vi "xcorr bkp nico.vi"(4 "shift":u8, 6 "N":u8, 7 "y":u32, 8 "x":u32, 9 "enable":bool, 10 "lag":u16) -> (1 "Rxy valid":bool, 2 "Rxy":u64, 3 "trigger":bool)   [LabVIEW 2017]
uses:
  <vilib>/rvi/FXPMathLib/basic elements/FxpDiscreteDelay/XNode/nifxpmath_DiscreteDelay.xnode
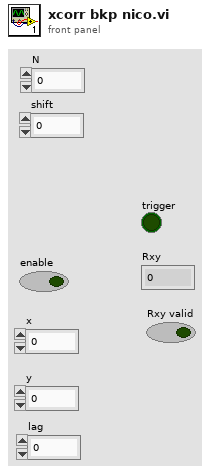
[diagram p1: front panel]
types:
  T1 = cluster{"Q":bool, "Q":bool, "Q":bool, "Q":bool, "valid":bool}
  T2 = cluster{"Q":bool, "Q":bool, "Q":bool, "Q":bool, "Q":bool, "Q":bool, "valid":bool}
  T3 = cluster{"Q":bool, "Q":bool, "Q":bool, "Q":bool, "Q":bool, "Q":bool, "Q":bool, "Q":bool, "Q":bool, "Q":bool, "Q":bool, "Q":bool, "valid":bool}
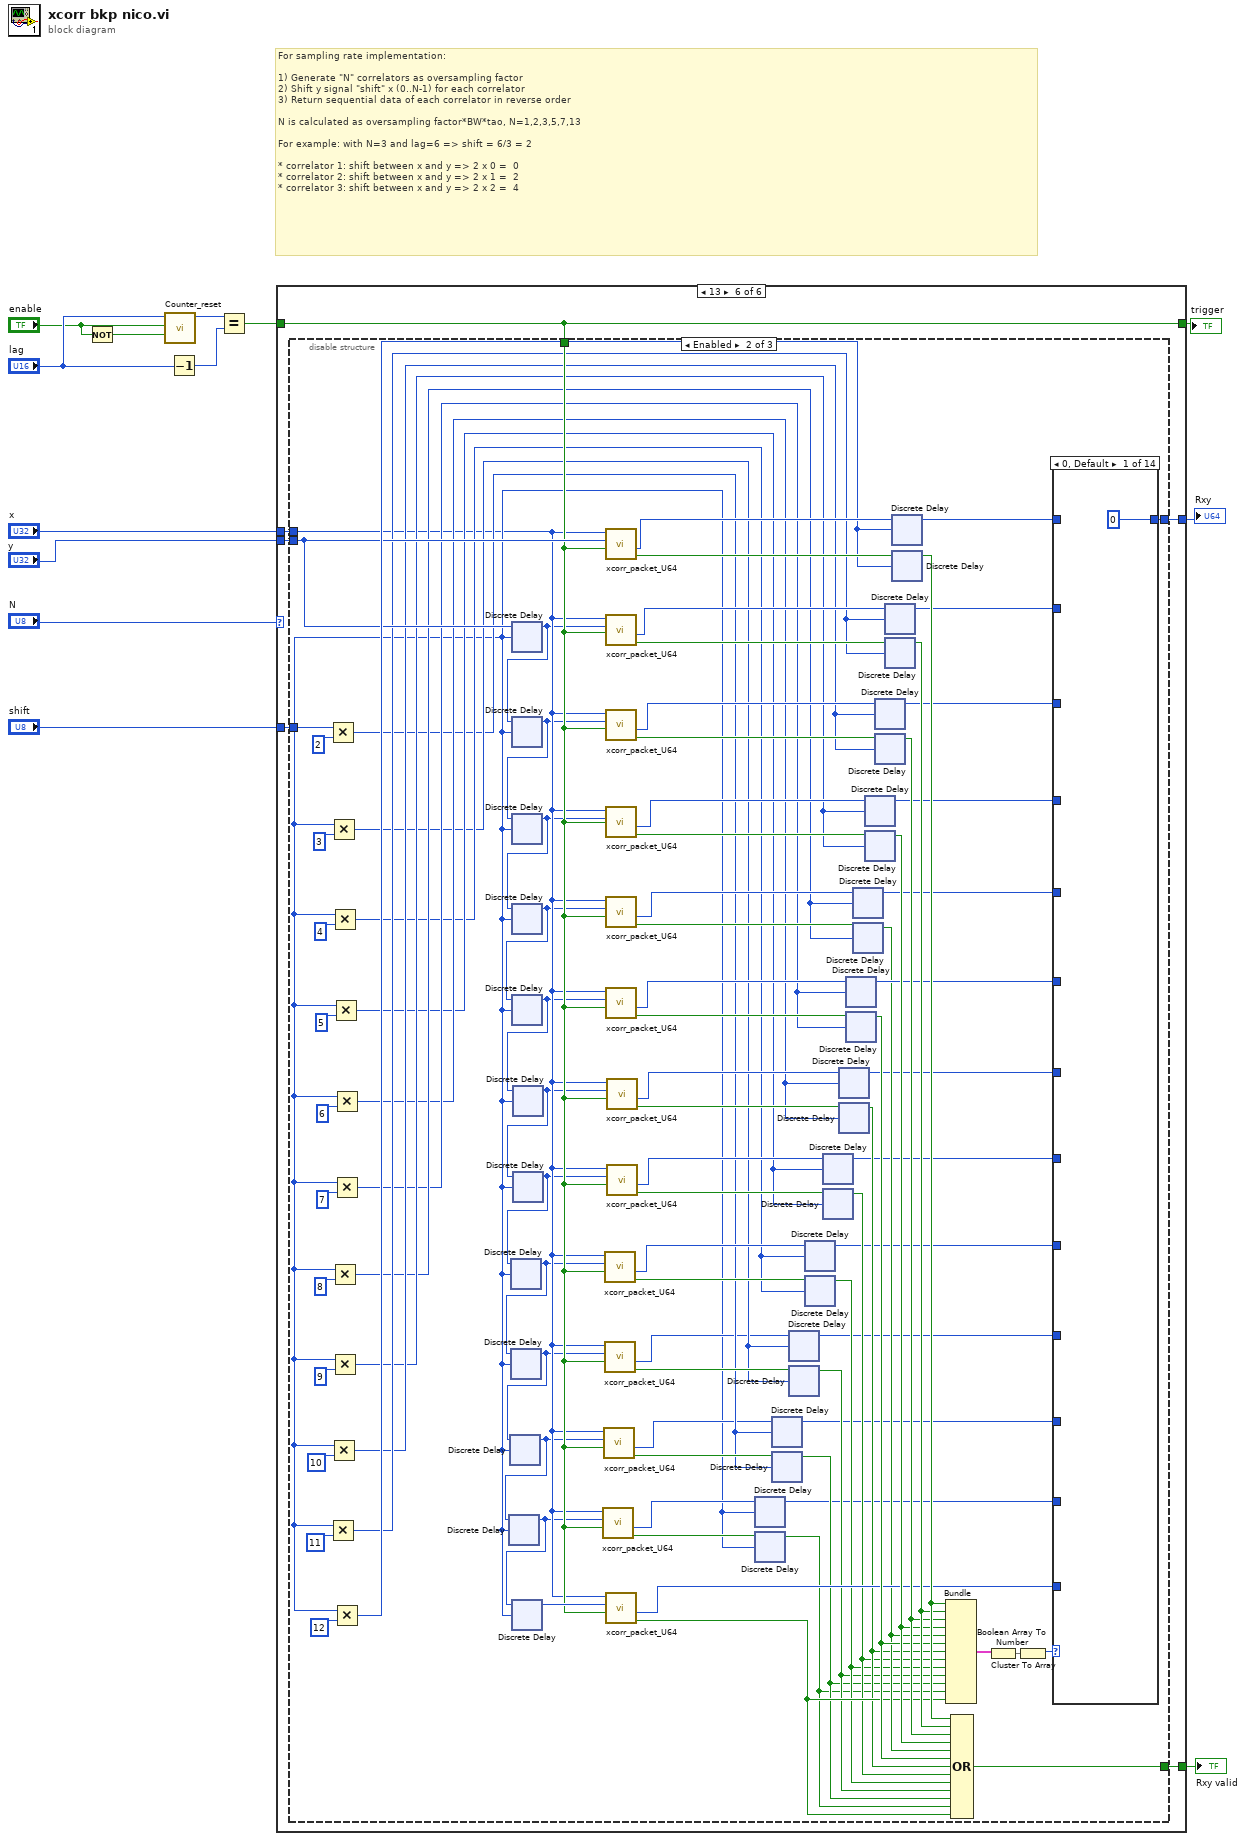
[diagram p0: block diagram]
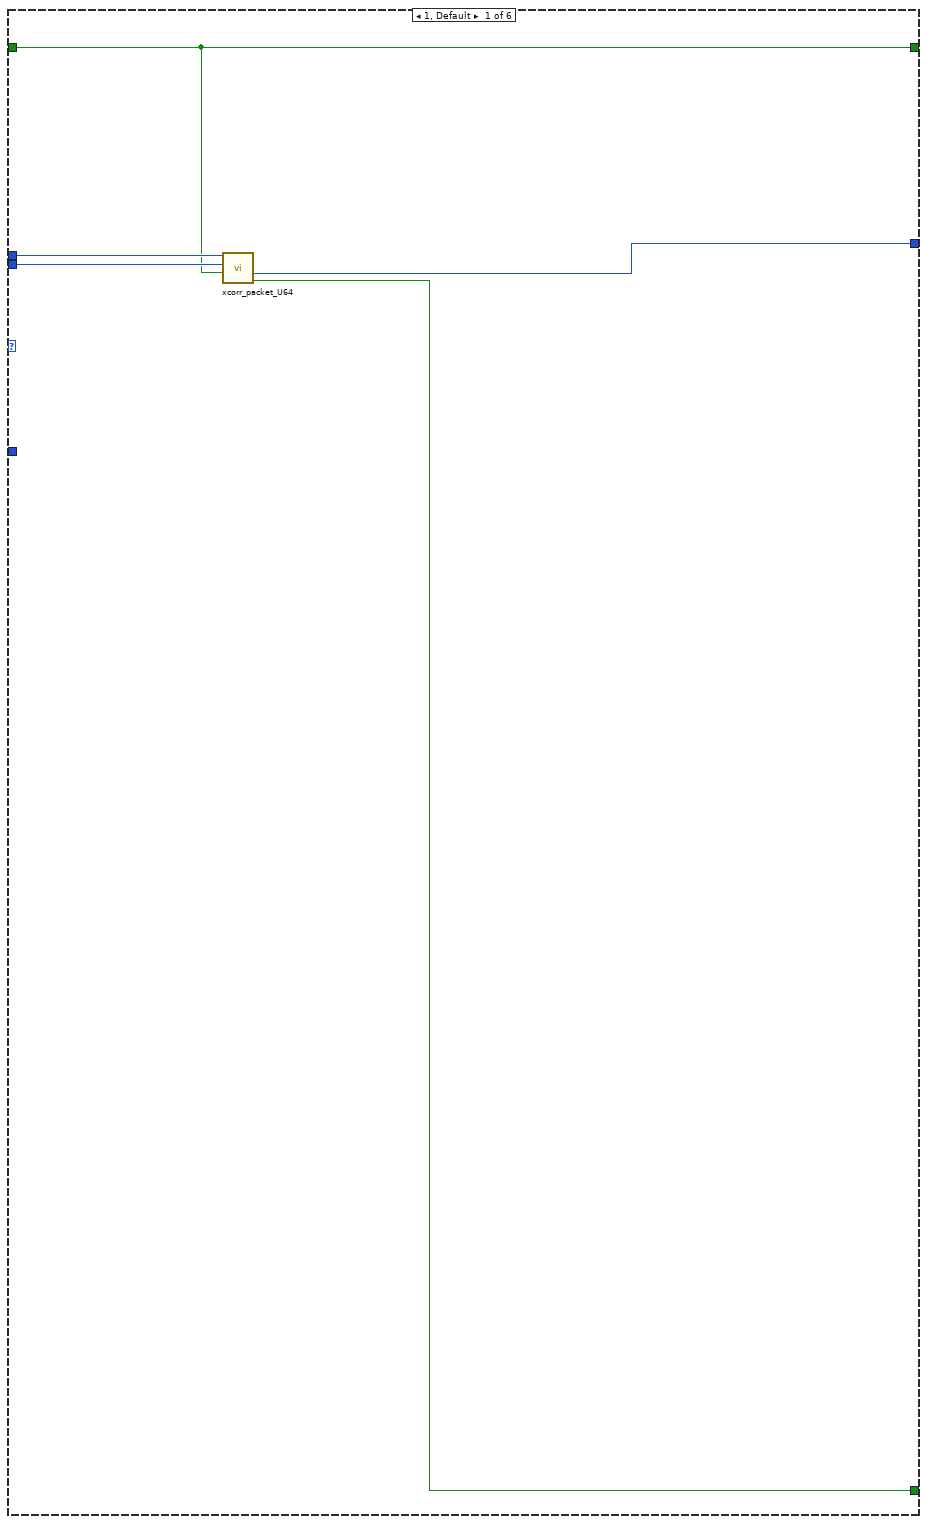
[diagram p2: hidden frame]
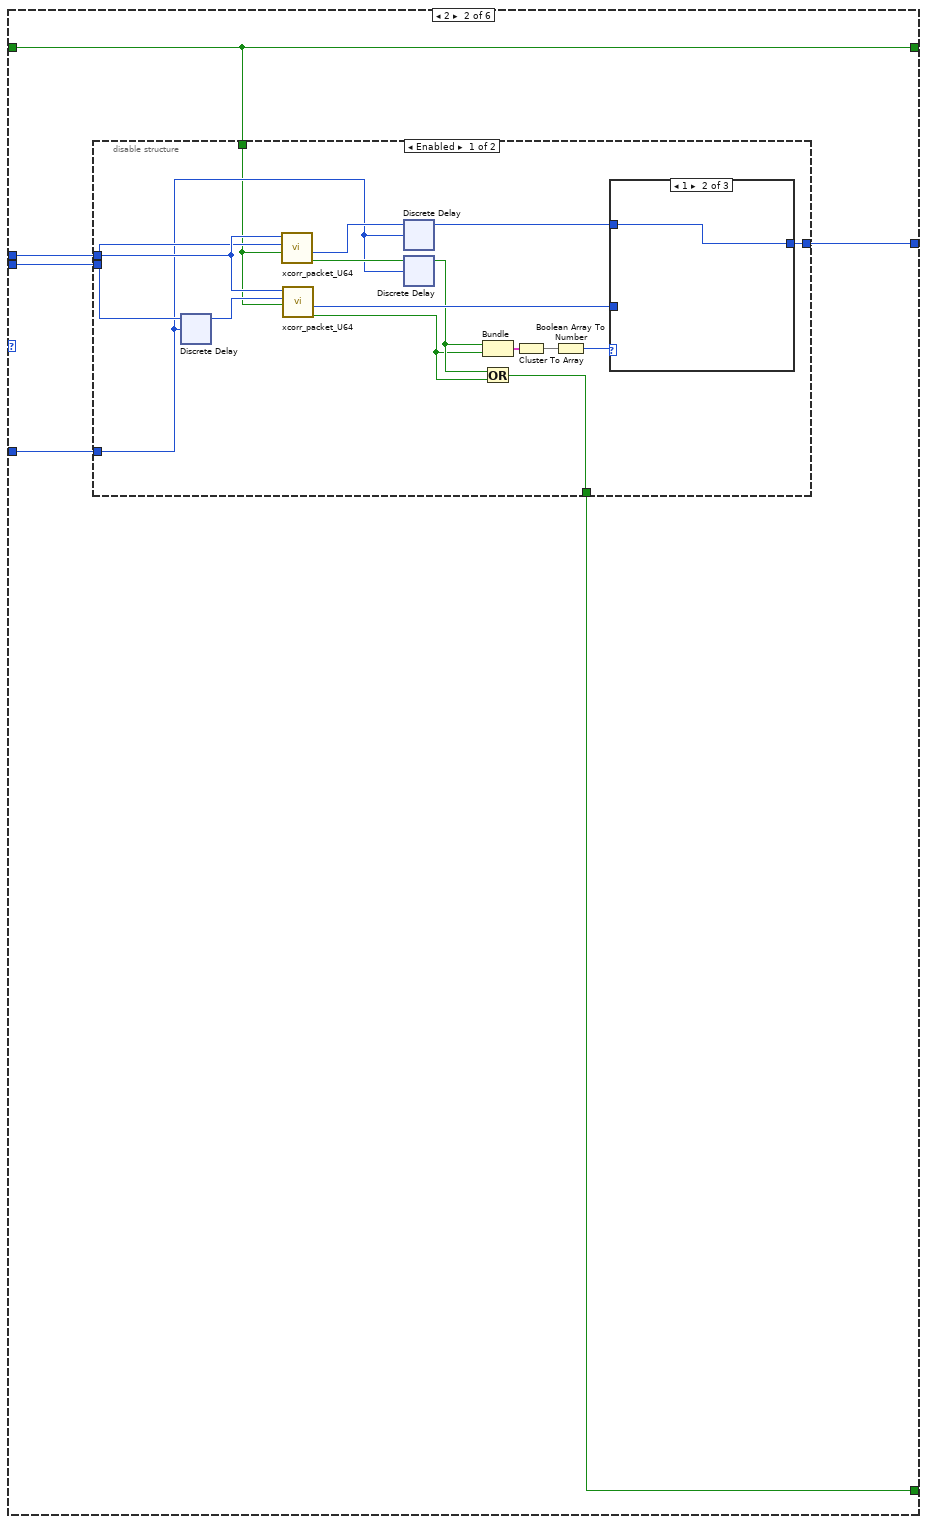
[diagram p3: hidden frame]
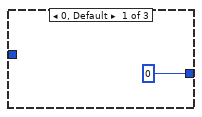
[diagram p4: hidden frame]
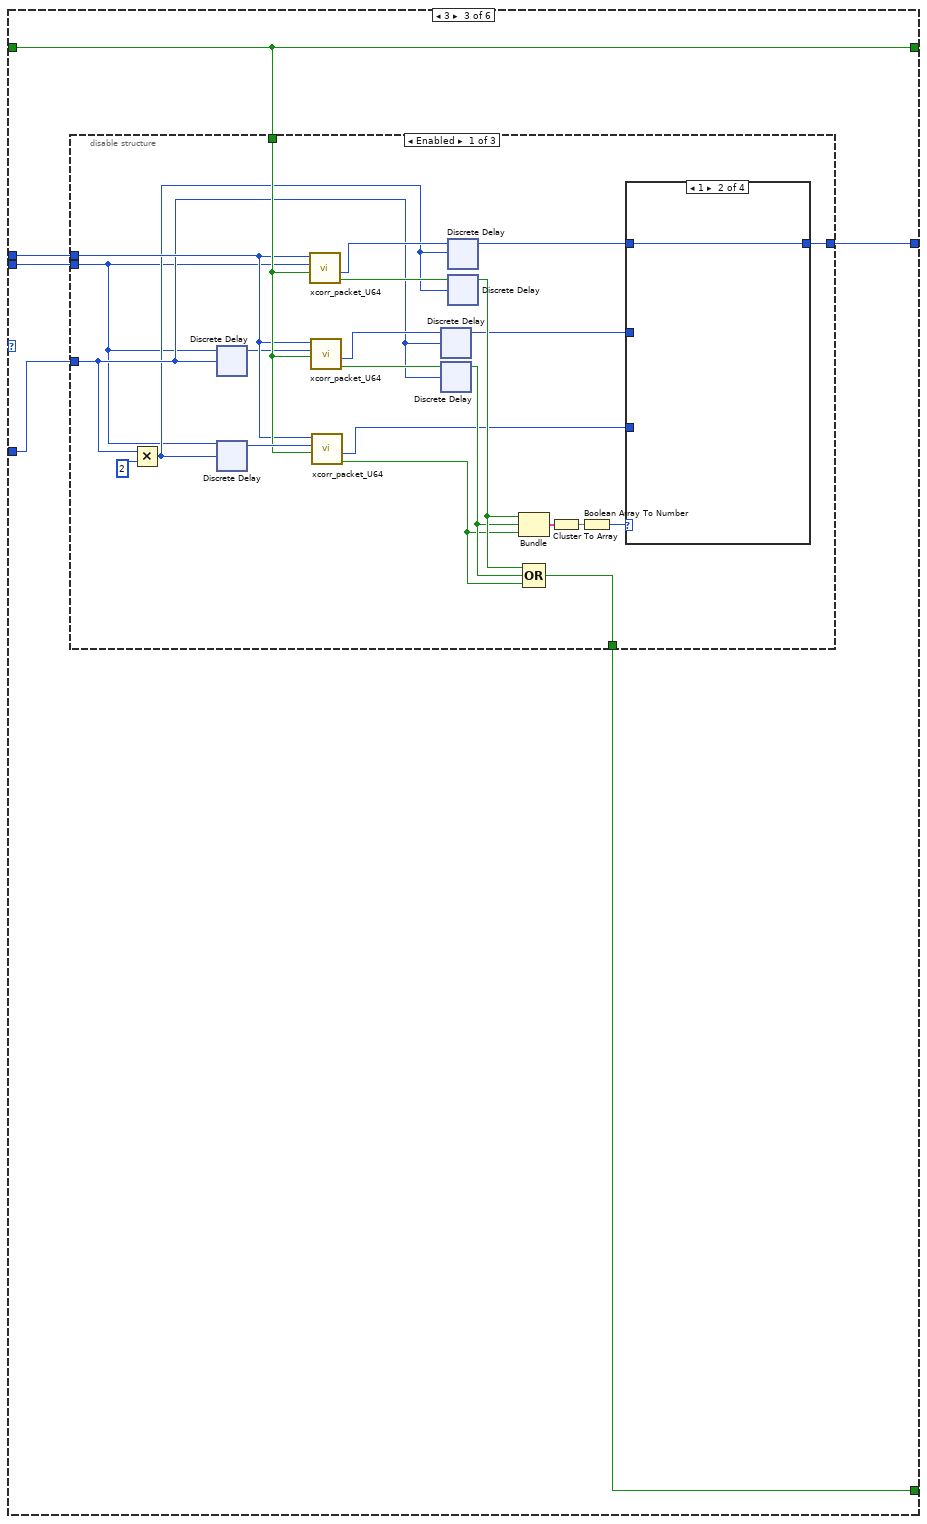
[diagram p7: hidden frame]
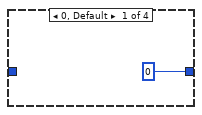
[diagram p8: hidden frame]
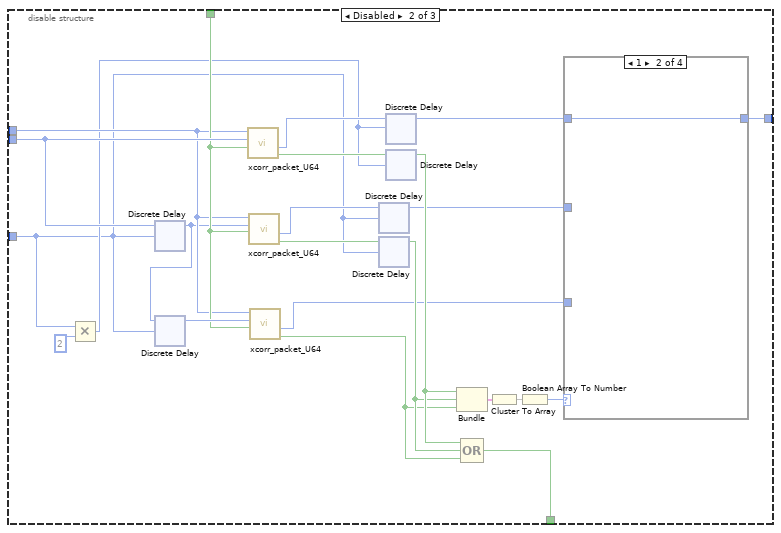
[diagram p11: hidden frame]
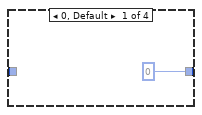
[diagram p12: hidden frame]
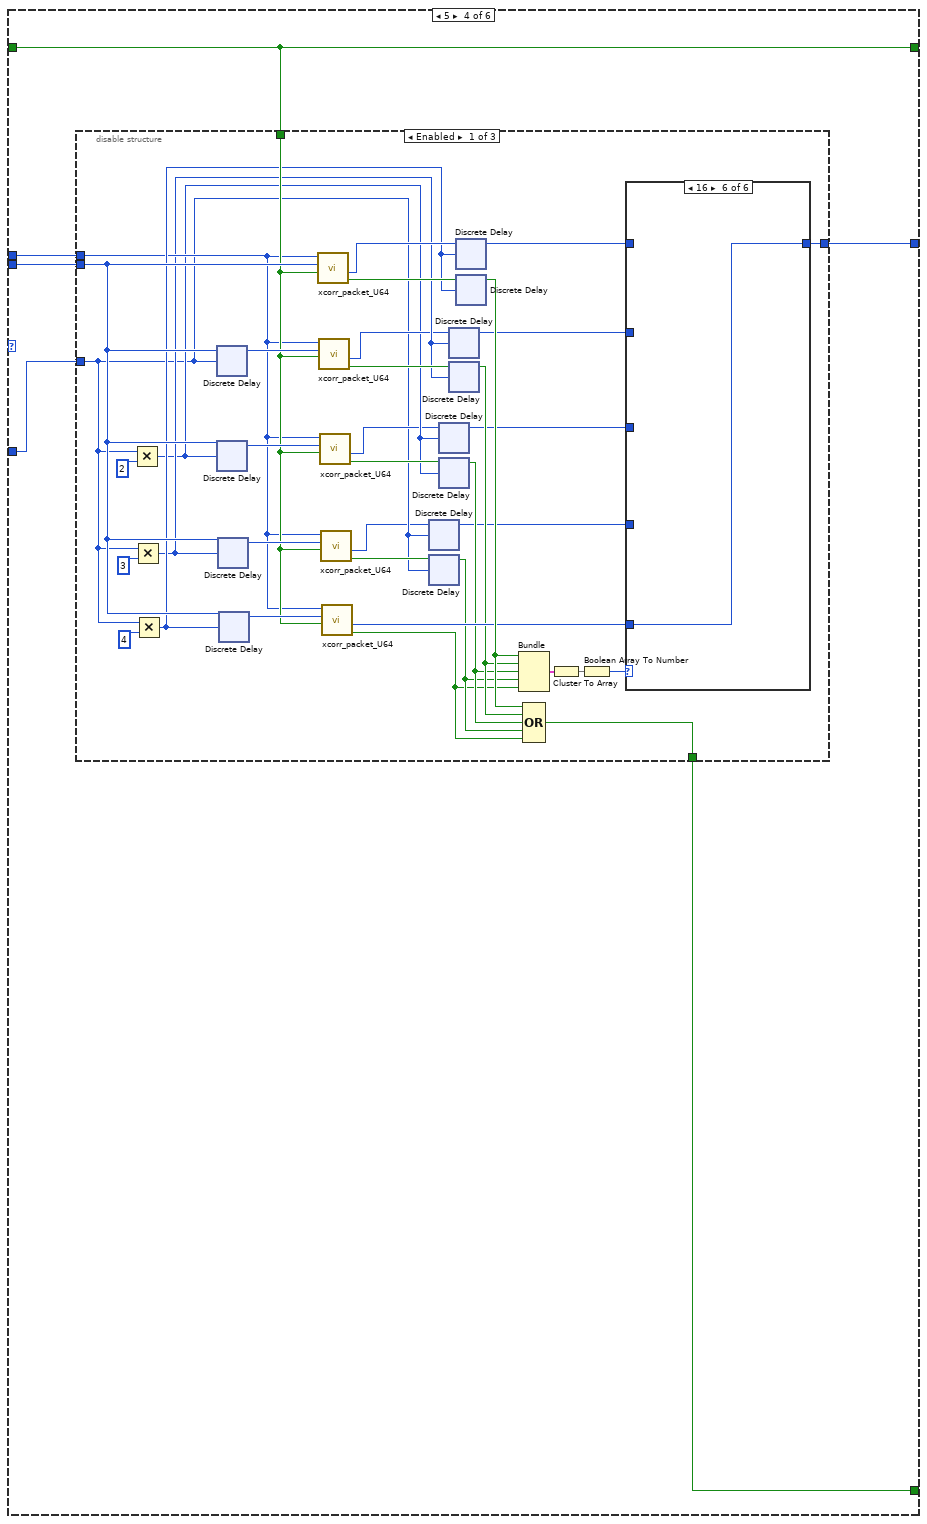
[diagram p16: hidden frame]
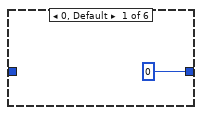
[diagram p17: hidden frame]
diagram:
  # "For sampling rate implementation:\n\n1) Generate \"N\" correlators as oversampling factor\n2) Shift y signal \"shift\" x (0..N-1) for each correlator\n3) Return sequential data of each correlator in reverse order\n\nN is calculated as oversampling factor*BW*tao, N=1,2,3,5,7,13\n\nFor example: with N=3 and lag=6 => shift = 6/3 = 2\n\n* correlator 1: shift between x and y => 2 x 0 =  0\n* correlator 2: shift between x and y => 2 x 1 =  2\n* correlator 3: shift between x and y => 2 x 2 =  4"
  n1 = Not(x="enable") -> (.not. x?=w10:bool)
  n2 = call "Counter_reset.vi"("reset"=w10, "enable"="enable", "limit"="lag") -> ("count"=w11:u16)  [unwired: 8 in]
  n3 = Decrement(x="lag") -> (x-1=w8:u16)
  n4 = Equal?(x=w11, y=w8) -> (x = y?=w3:bool)
  n5 = case shown="13" "N" {
    tunnel: [w14 w19 w48 w108 w200 w324] -> w7
    tunnel: [w18 w23 w49 w109 w201 w325] -> w13
    tunnel: [w15 w20 w46 w106 w196 w321] -> w12
    tunnel: w3 -> [w15 w20 w46 w106 w196 w321]
    tunnel: "x" -> [w17 w24 w45 w105 w197 w322]
    tunnel: "y" -> [w16 w22 w47 w107 w199 w323]
    tunnel: "shift" -> [_ w21 w44 w104 w198 w320]
    frame 1, Default {
      n6 = call "xcorr_packet_U64.vi"("x"=w17, "y"=w16, "trigger"=w15) -> ("out"=w14:u64, "valid"=w18:bool)  [unwired: 5 in]
    }
    frame 2 {
      n7 = disable-structure shown="Enabled" {
        disable-tunnel: w24 -> [w40 _]
        disable-tunnel: [w39 _] -> w23
        disable-tunnel: w22 -> [w38 _]
        disable-tunnel: w21 -> [w34 _]
        disable-tunnel: w20 -> [w33 _]
        disable-tunnel: [w27 _] -> w19
        frame Enabled {
          n8 = xnode ("Discrete Delay")("D"=w38, "n-1[0..255]"=w34) -> ("Q"=w37:u32)
          n9 = call "xcorr_packet_U64.vi"("x"=w40, "y"=w38, "trigger"=w33) -> ("out"=w36:u64, "valid"=w35:bool)  [unwired: 5 in]
          n10 = call "xcorr_packet_U64.vi"("x"=w40, "y"=w37, "trigger"=w33) -> ("out"=w28:u64, "valid"=w25:bool)  [unwired: 5 in]
          n11 = xnode ("Discrete Delay")("D"=w36, "n-1[0..255]"=w34) -> ("Q"=w29:u64)
          n12 = xnode ("Discrete Delay")("D"=w35, "n-1[0..255]"=w34) -> ("Q"=w26:bool)
          n13 = Bundle("Q"=w26, "valid"=w25) -> (w32:cluster{"Q":bool, "valid":bool})  [unwired: 1 in]
          n14 = Or(x=w26, y=w25) -> (x .or. y?=w39:bool)
          n15 = Cluster To Array(cluster=w32) -> (array=w31:bool[])
          n16 = Boolean Array To Number(Boolean array=w31) -> (number=w30:u8)
          n17 = case shown="1" w30 {
            tunnel: [u64 0 ("out") w42 w43] -> w27
            tunnel: w29 -> [_ w42 _]
            tunnel: w28 -> [_ _ w43]
            frame 0, Default {
            }
            frame 1 {
            }
            frame 2 {
            }
          }
        }
        frame Disabled {
        }
      }
    }
    frame 3 {
      n18 = disable-structure shown="Enabled" {
        disable-tunnel: [w72 w99 _] -> w49
        disable-tunnel: [w67 w94 _] -> w48
        disable-tunnel: w47 -> [w50 w91 _]
        disable-tunnel: w46 -> [w64 w90 _]
        disable-tunnel: w45 -> [w60 w86 _]
        disable-tunnel: w44 -> [w53 w78 _]
        frame Enabled {
          n19 = Multiply(x=w53, y=u8 2 ("x")) -> (x*y=w51:u8)
          n20 = xnode ("Discrete Delay")("D"=w50, "n-1[0..255]"=w53) -> ("Q"=w52:u32)
          n21 = xnode ("Discrete Delay")("D"=w50, "n-1[0..255]"=w51) -> ("Q"=w65:u32)
          n22 = call "xcorr_packet_U64.vi"("x"=w60, "y"=w50, "trigger"=w64) -> ("out"=w71:u64, "valid"=w70:bool)  [unwired: 5 in]
          n23 = call "xcorr_packet_U64.vi"("x"=w60, "y"=w52, "trigger"=w64) -> ("out"=w59:u64, "valid"=w61:bool)  [unwired: 5 in]
          n24 = call "xcorr_packet_U64.vi"("x"=w60, "y"=w65, "trigger"=w64) -> ("out"=w54:u64, "valid"=w55:bool)  [unwired: 5 in]
          n25 = xnode ("Discrete Delay")("D"=w59, "n-1[0..255]"=w53) -> ("Q"=w58:u64)
          n26 = xnode ("Discrete Delay")("D"=w61, "n-1[0..255]"=w53) -> ("Q"=w62:bool)
          n27 = xnode ("Discrete Delay")("D"=w71, "n-1[0..255]"=w51) -> ("Q"=w68:u64)
          n28 = xnode ("Discrete Delay")("D"=w70, "n-1[0..255]"=w51) -> ("Q"=w63:bool)
          n29 = Bundle("Q"=w63, "Q"=w62, "valid"=w55) -> (w57:cluster{"Q":bool, "Q":bool, "valid":bool})  [unwired: 1 in]
          n30 = Compound Arithmetic op=OR(w63, w62, w55) -> (w72:bool)
          n31 = Cluster To Array(cluster=w57) -> (array=w56:bool[])
          n32 = Boolean Array To Number(Boolean array=w56) -> (number=w69:u8)
          n33 = case shown="1" w69 {
            tunnel: [u64 0 ("out") w74 w75 w76] -> w67
            tunnel: w68 -> [_ w74 _ _]
            tunnel: w58 -> [_ _ w75 _]
            tunnel: w54 -> [_ _ _ w76]
            frame 0, Default {
            }
            frame 1 {
            }
            frame 2 {
            }
            frame 4 {
            }
          }
        }
        frame Disabled {
          n34 = Multiply(x=w78, y=u8 2 ("x")) -> (x*y=w83:u8)
          n35 = xnode ("Discrete Delay")("D"=w91, "n-1[0..255]"=w78) -> ("Q"=w77:u32)
          n36 = xnode ("Discrete Delay")("D"=w77, "n-1[0..255]"=w78) -> ("Q"=w92:u32)
          n37 = call "xcorr_packet_U64.vi"("x"=w86, "y"=w91, "trigger"=w90) -> ("out"=w98:u64, "valid"=w97:bool)  [unwired: 5 in]
          n38 = call "xcorr_packet_U64.vi"("x"=w86, "y"=w77, "trigger"=w90) -> ("out"=w85:u64, "valid"=w87:bool)  [unwired: 5 in]
          n39 = call "xcorr_packet_U64.vi"("x"=w86, "y"=w92, "trigger"=w90) -> ("out"=w79:u64, "valid"=w80:bool)  [unwired: 5 in]
          n40 = xnode ("Discrete Delay")("D"=w85, "n-1[0..255]"=w78) -> ("Q"=w84:u64)
          n41 = xnode ("Discrete Delay")("D"=w87, "n-1[0..255]"=w78) -> ("Q"=w88:bool)
          n42 = xnode ("Discrete Delay")("D"=w98, "n-1[0..255]"=w83) -> ("Q"=w95:u64)
          n43 = xnode ("Discrete Delay")("D"=w97, "n-1[0..255]"=w83) -> ("Q"=w89:bool)
          n44 = Bundle("Q"=w89, "Q"=w88, "valid"=w80) -> (w82:cluster{"Q":bool, "Q":bool, "valid":bool})  [unwired: 1 in]
          n45 = Compound Arithmetic op=OR(w89, w88, w80) -> (w99:bool)
          n46 = Cluster To Array(cluster=w82) -> (array=w81:bool[])
          n47 = Boolean Array To Number(Boolean array=w81) -> (number=w96:u8)
          n48 = case shown="1" w96 {
            tunnel: [u64 0 ("out") w101 w102 w103] -> w94
            tunnel: w95 -> [_ w101 _ _]
            tunnel: w84 -> [_ _ w102 _]
            tunnel: w79 -> [_ _ _ w103]
            frame 0, Default {
            }
            frame 1 {
            }
            frame 2 {
            }
            frame 4 {
            }
          }
        }
        frame Disabled {
        }
      }
    }
    frame 5 {
      n49 = disable-structure shown="Enabled" {
        disable-tunnel: [w146 w189 _] -> w109
        disable-tunnel: [w138 w182 _] -> w108
        disable-tunnel: w107 -> [w131 w177 _]
        disable-tunnel: w106 -> [w130 w176 _]
        disable-tunnel: w105 -> [w120 w166 _]
        disable-tunnel: w104 -> [w112 w156 _]
        frame Enabled {
          n50 = Multiply(x=w112, y=u8 2 ("x")) -> (x*y=w115:u8)
          n51 = Multiply(x=w112, y=u8 3 ("x")) -> (x*y=w118:u8)
          n52 = Multiply(x=w112, y=u8 4 ("x")) -> (x*y=w127:u8)
          n53 = xnode ("Discrete Delay")("D"=w131, "n-1[0..255]"=w112) -> ("Q"=w145:u32)
          n54 = xnode ("Discrete Delay")("D"=w131, "n-1[0..255]"=w115) -> ("Q"=w136:u32)
          n55 = xnode ("Discrete Delay")("D"=w131, "n-1[0..255]"=w118) -> ("Q"=w134:u32)
          n56 = xnode ("Discrete Delay")("D"=w131, "n-1[0..255]"=w127) -> ("Q"=w132:u32)
          n57 = call "xcorr_packet_U64.vi"("x"=w120, "y"=w131, "trigger"=w130) -> ("out"=w144:u64, "valid"=w143:bool)  [unwired: 5 in]
          n58 = call "xcorr_packet_U64.vi"("x"=w120, "y"=w145, "trigger"=w130) -> ("out"=w117:u64, "valid"=w125:bool)  [unwired: 5 in]
          n59 = call "xcorr_packet_U64.vi"("x"=w120, "y"=w136, "trigger"=w130) -> ("out"=w114:u64, "valid"=w124:bool)  [unwired: 5 in]
          n60 = call "xcorr_packet_U64.vi"("x"=w120, "y"=w134, "trigger"=w130) -> ("out"=w111:u64, "valid"=w122:bool)  [unwired: 5 in]
          n61 = call "xcorr_packet_U64.vi"("x"=w120, "y"=w132, "trigger"=w130) -> ("out"=w128:u64, "valid"=w119:bool)  [unwired: 5 in]
          n62 = xnode ("Discrete Delay")("D"=w111, "n-1[0..255]"=w112) -> ("Q"=w110:u64)
          n63 = xnode ("Discrete Delay")("D"=w122, "n-1[0..255]"=w112) -> ("Q"=w121:bool)
          n64 = xnode ("Discrete Delay")("D"=w114, "n-1[0..255]"=w115) -> ("Q"=w113:u64)
          n65 = xnode ("Discrete Delay")("D"=w124, "n-1[0..255]"=w115) -> ("Q"=w123:bool)
          n66 = xnode ("Discrete Delay")("D"=w117, "n-1[0..255]"=w118) -> ("Q"=w116:u64)
          n67 = xnode ("Discrete Delay")("D"=w125, "n-1[0..255]"=w118) -> ("Q"=w126:bool)
          n68 = xnode ("Discrete Delay")("D"=w144, "n-1[0..255]"=w127) -> ("Q"=w139:u64)
          n69 = xnode ("Discrete Delay")("D"=w143, "n-1[0..255]"=w127) -> ("Q"=w129:bool)
          n70 = Bundle("Q"=w129, "Q"=w126, "Q"=w123, "Q"=w121, "valid"=w119) -> (w142:T1)  [unwired: 1 in]
          n71 = Compound Arithmetic op=OR(w129, w126, w123, w121, w119) -> (w146:bool)
          n72 = Cluster To Array(cluster=w142) -> (array=w141:bool[])
          n73 = Boolean Array To Number(Boolean array=w141) -> (number=w140:u8)
          n74 = case shown="16" w140 {
            tunnel: [u64 0 ("out") w148 w149 w150 w151 w152] -> w138
            tunnel: w139 -> [_ w148 _ _ _ _]
            tunnel: w116 -> [_ _ w149 _ _ _]
            tunnel: w113 -> [_ _ _ w150 _ _]
            tunnel: w110 -> [_ _ _ _ w151 _]
            tunnel: w128 -> [_ _ _ _ _ w152]
            frame 0, Default {
            }
            frame 1 {
            }
            frame 2 {
            }
            frame 4 {
            }
            frame 8 {
            }
            frame 16 {
            }
          }
        }
        frame Disabled {
          n75 = Multiply(x=w156, y=u8 2 ("x")) -> (x*y=w161:u8)
          n76 = Multiply(x=w156, y=u8 3 ("x")) -> (x*y=w164:u8)
          n77 = Multiply(x=w156, y=u8 4 ("x")) -> (x*y=w173:u8)
          n78 = xnode ("Discrete Delay")("D"=w177, "n-1[0..255]"=w156) -> ("Q"=w155:u32)
          n79 = xnode ("Discrete Delay")("D"=w155, "n-1[0..255]"=w156) -> ("Q"=w154:u32)
          n80 = xnode ("Discrete Delay")("D"=w154, "n-1[0..255]"=w156) -> ("Q"=w153:u32)
          n81 = xnode ("Discrete Delay")("D"=w153, "n-1[0..255]"=w156) -> ("Q"=w178:u32)
          n82 = call "xcorr_packet_U64.vi"("x"=w166, "y"=w177, "trigger"=w176) -> ("out"=w188:u64, "valid"=w187:bool)  [unwired: 5 in]
          n83 = call "xcorr_packet_U64.vi"("x"=w166, "y"=w155, "trigger"=w176) -> ("out"=w163:u64, "valid"=w171:bool)  [unwired: 5 in]
          n84 = call "xcorr_packet_U64.vi"("x"=w166, "y"=w154, "trigger"=w176) -> ("out"=w160:u64, "valid"=w170:bool)  [unwired: 5 in]
          n85 = call "xcorr_packet_U64.vi"("x"=w166, "y"=w153, "trigger"=w176) -> ("out"=w158:u64, "valid"=w168:bool)  [unwired: 5 in]
          n86 = call "xcorr_packet_U64.vi"("x"=w166, "y"=w178, "trigger"=w176) -> ("out"=w174:u64, "valid"=w165:bool)  [unwired: 5 in]
          n87 = xnode ("Discrete Delay")("D"=w158, "n-1[0..255]"=w156) -> ("Q"=w157:u64)
          n88 = xnode ("Discrete Delay")("D"=w168, "n-1[0..255]"=w156) -> ("Q"=w167:bool)
          n89 = xnode ("Discrete Delay")("D"=w160, "n-1[0..255]"=w161) -> ("Q"=w159:u64)
          n90 = xnode ("Discrete Delay")("D"=w170, "n-1[0..255]"=w161) -> ("Q"=w169:bool)
          n91 = xnode ("Discrete Delay")("D"=w163, "n-1[0..255]"=w164) -> ("Q"=w162:u64)
          n92 = xnode ("Discrete Delay")("D"=w171, "n-1[0..255]"=w164) -> ("Q"=w172:bool)
          n93 = xnode ("Discrete Delay")("D"=w188, "n-1[0..255]"=w173) -> ("Q"=w183:u64)
          n94 = xnode ("Discrete Delay")("D"=w187, "n-1[0..255]"=w173) -> ("Q"=w175:bool)
          n95 = Bundle("Q"=w175, "Q"=w172, "Q"=w169, "Q"=w167, "valid"=w165) -> (w186:T1)  [unwired: 1 in]
          n96 = Compound Arithmetic op=OR(w175, w172, w169, w167, w165) -> (w189:bool)
          n97 = Cluster To Array(cluster=w186) -> (array=w185:bool[])
          n98 = Boolean Array To Number(Boolean array=w185) -> (number=w184:u8)
          n99 = case shown="16" w184 {
            tunnel: [u64 0 ("out") w191 w192 w193 w194 w195] -> w182
            tunnel: w183 -> [_ w191 _ _ _ _]
            tunnel: w162 -> [_ _ w192 _ _ _]
            tunnel: w159 -> [_ _ _ w193 _ _]
            tunnel: w157 -> [_ _ _ _ w194 _]
            tunnel: w174 -> [_ _ _ _ _ w195]
            frame 0, Default {
            }
            frame 1 {
            }
            frame 2 {
            }
            frame 4 {
            }
            frame 8 {
            }
            frame 16 {
            }
          }
        }
        frame Disabled {
        }
      }
    }
    frame 7 {
      n100 = disable-structure shown="Enabled" {
        disable-tunnel: [w252 w311 _] -> w201
        disable-tunnel: [w245 w305 _] -> w200
        disable-tunnel: w199 -> [w211 w275 _]
        disable-tunnel: w198 -> [w210 w266 _]
        disable-tunnel: w197 -> [w209 w274 _]
        disable-tunnel: w196 -> [w208 w273 _]
        frame Disabled {
          n101 = Multiply(x=w210, y=u8 2 ("x")) -> (x*y=w214:u8)
          n102 = Multiply(x=w210, y=u8 3 ("x")) -> (x*y=w215:u8)
          n103 = Multiply(x=w210, y=u8 4 ("x")) -> (x*y=w216:u8)
          n104 = Multiply(x=w210, y=u8 5 ("x")) -> (x*y=w217:u8)
          n105 = Multiply(x=w210, y=u8 6 ("x")) -> (x*y=w205:u8)
          n106 = xnode ("Discrete Delay")("D"=w211, "n-1[0..255]"=w210) -> ("Q"=w251:u32)
          n107 = xnode ("Discrete Delay")("D"=w211, "n-1[0..255]"=w214) -> ("Q"=w243:u32)
          n108 = xnode ("Discrete Delay")("D"=w211, "n-1[0..255]"=w215) -> ("Q"=w241:u32)
          n109 = xnode ("Discrete Delay")("D"=w211, "n-1[0..255]"=w216) -> ("Q"=w239:u32)
          n110 = xnode ("Discrete Delay")("D"=w211, "n-1[0..255]"=w217) -> ("Q"=w224:u32)
          n111 = xnode ("Discrete Delay")("D"=w211, "n-1[0..255]"=w205) -> ("Q"=w212:u32)
          n112 = call "xcorr_packet_U64.vi"("x"=w209, "y"=w211, "trigger"=w208) -> ("out"=w250:u64, "valid"=w249:bool)  [unwired: 5 in]
          n113 = call "xcorr_packet_U64.vi"("x"=w209, "y"=w251, "trigger"=w208) -> ("out"=w231:u64, "valid"=w236:bool)  [unwired: 5 in]
          n114 = call "xcorr_packet_U64.vi"("x"=w209, "y"=w243, "trigger"=w208) -> ("out"=w229:u64, "valid"=w235:bool)  [unwired: 5 in]
          n115 = call "xcorr_packet_U64.vi"("x"=w209, "y"=w241, "trigger"=w208) -> ("out"=w227:u64, "valid"=w233:bool)  [unwired: 5 in]
          n116 = call "xcorr_packet_U64.vi"("x"=w209, "y"=w239, "trigger"=w208) -> ("out"=w219:u64, "valid"=w203:bool)  [unwired: 5 in]
          n117 = call "xcorr_packet_U64.vi"("x"=w209, "y"=w224, "trigger"=w208) -> ("out"=w221:u64, "valid"=w223:bool)  [unwired: 5 in]
          n118 = call "xcorr_packet_U64.vi"("x"=w209, "y"=w212, "trigger"=w208) -> ("out"=w204:u64, "valid"=w207:bool)  [unwired: 5 in]
          n119 = xnode ("Discrete Delay")("D"=w221, "n-1[0..255]"=w210) -> ("Q"=w220:u64)
          n120 = xnode ("Discrete Delay")("D"=w223, "n-1[0..255]"=w210) -> ("Q"=w222:bool)
          n121 = xnode ("Discrete Delay")("D"=w219, "n-1[0..255]"=w214) -> ("Q"=w218:u64)
          n122 = xnode ("Discrete Delay")("D"=w203, "n-1[0..255]"=w214) -> ("Q"=w202:bool)
          n123 = xnode ("Discrete Delay")("D"=w227, "n-1[0..255]"=w215) -> ("Q"=w226:u64)
          n124 = xnode ("Discrete Delay")("D"=w233, "n-1[0..255]"=w215) -> ("Q"=w232:bool)
          n125 = xnode ("Discrete Delay")("D"=w229, "n-1[0..255]"=w216) -> ("Q"=w228:u64)
          n126 = xnode ("Discrete Delay")("D"=w235, "n-1[0..255]"=w216) -> ("Q"=w234:bool)
          n127 = xnode ("Discrete Delay")("D"=w231, "n-1[0..255]"=w217) -> ("Q"=w230:u64)
          n128 = xnode ("Discrete Delay")("D"=w236, "n-1[0..255]"=w217) -> ("Q"=w237:bool)
          n129 = xnode ("Discrete Delay")("D"=w250, "n-1[0..255]"=w205) -> ("Q"=w246:u64)
          n130 = xnode ("Discrete Delay")("D"=w249, "n-1[0..255]"=w205) -> ("Q"=w238:bool)
          n131 = Bundle("Q"=w238, "Q"=w237, "Q"=w234, "Q"=w232, "Q"=w202, "Q"=w222, "valid"=w207) -> (w206:T2)  [unwired: 1 in]
          n132 = Compound Arithmetic op=OR(w238, w237, w234, w232, w202, w222, w207) -> (w252:bool)
          n133 = Cluster To Array(cluster=w206) -> (array=w248:bool[])
          n134 = Boolean Array To Number(Boolean array=w248) -> (number=w247:u8)
          n135 = case shown="32" w247 {
            tunnel: [u64 0 ("out") w254 w255 w256 w257 w258 w259 w260] -> w245
            tunnel: w246 -> [_ w254 _ _ _ _ _ _]
            tunnel: w230 -> [_ _ w255 _ _ _ _ _]
            tunnel: w228 -> [_ _ _ w256 _ _ _ _]
            tunnel: w226 -> [_ _ _ _ w257 _ _ _]
            tunnel: w218 -> [_ _ _ _ _ w258 _ _]
            tunnel: w220 -> [_ _ _ _ _ _ w259 _]
            tunnel: w204 -> [_ _ _ _ _ _ _ w260]
            frame 0, Default {
            }
            frame 1 {
            }
            frame 2 {
            }
            frame 4 {
            }
            frame 8 {
            }
            frame 16 {
            }
            frame 32 {
            }
            frame 64 {
            }
          }
        }
        frame Enabled {
          n136 = Multiply(x=w266, y=u8 2 ("x")) -> (x*y=w278:u8)
          n137 = Multiply(x=w266, y=u8 3 ("x")) -> (x*y=w279:u8)
          n138 = Multiply(x=w266, y=u8 4 ("x")) -> (x*y=w280:u8)
          n139 = Multiply(x=w266, y=u8 5 ("x")) -> (x*y=w281:u8)
          n140 = Multiply(x=w266, y=u8 6 ("x")) -> (x*y=w270:u8)
          n141 = xnode ("Discrete Delay")("D"=w275, "n-1[0..255]"=w266) -> ("Q"=w265:u32)
          n142 = xnode ("Discrete Delay")("D"=w265, "n-1[0..255]"=w266) -> ("Q"=w264:u32)
          n143 = xnode ("Discrete Delay")("D"=w264, "n-1[0..255]"=w266) -> ("Q"=w263:u32)
          n144 = xnode ("Discrete Delay")("D"=w263, "n-1[0..255]"=w266) -> ("Q"=w262:u32)
          n145 = xnode ("Discrete Delay")("D"=w262, "n-1[0..255]"=w266) -> ("Q"=w261:u32)
          n146 = xnode ("Discrete Delay")("D"=w261, "n-1[0..255]"=w266) -> ("Q"=w276:u32)
          n147 = call "xcorr_packet_U64.vi"("x"=w274, "y"=w275, "trigger"=w273) -> ("out"=w310:u64, "valid"=w309:bool)  [unwired: 5 in]
          n148 = call "xcorr_packet_U64.vi"("x"=w274, "y"=w265, "trigger"=w273) -> ("out"=w294:u64, "valid"=w299:bool)  [unwired: 5 in]
          n149 = call "xcorr_packet_U64.vi"("x"=w274, "y"=w264, "trigger"=w273) -> ("out"=w292:u64, "valid"=w298:bool)  [unwired: 5 in]
          n150 = call "xcorr_packet_U64.vi"("x"=w274, "y"=w263, "trigger"=w273) -> ("out"=w290:u64, "valid"=w296:bool)  [unwired: 5 in]
          n151 = call "xcorr_packet_U64.vi"("x"=w274, "y"=w262, "trigger"=w273) -> ("out"=w283:u64, "valid"=w268:bool)  [unwired: 5 in]
          n152 = call "xcorr_packet_U64.vi"("x"=w274, "y"=w261, "trigger"=w273) -> ("out"=w285:u64, "valid"=w287:bool)  [unwired: 5 in]
          n153 = call "xcorr_packet_U64.vi"("x"=w274, "y"=w276, "trigger"=w273) -> ("out"=w269:u64, "valid"=w272:bool)  [unwired: 5 in]
          n154 = xnode ("Discrete Delay")("D"=w285, "n-1[0..255]"=w266) -> ("Q"=w284:u64)
          n155 = xnode ("Discrete Delay")("D"=w287, "n-1[0..255]"=w266) -> ("Q"=w286:bool)
          n156 = xnode ("Discrete Delay")("D"=w283, "n-1[0..255]"=w278) -> ("Q"=w282:u64)
          n157 = xnode ("Discrete Delay")("D"=w268, "n-1[0..255]"=w278) -> ("Q"=w267:bool)
          n158 = xnode ("Discrete Delay")("D"=w290, "n-1[0..255]"=w279) -> ("Q"=w289:u64)
          n159 = xnode ("Discrete Delay")("D"=w296, "n-1[0..255]"=w279) -> ("Q"=w295:bool)
          n160 = xnode ("Discrete Delay")("D"=w292, "n-1[0..255]"=w280) -> ("Q"=w291:u64)
          n161 = xnode ("Discrete Delay")("D"=w298, "n-1[0..255]"=w280) -> ("Q"=w297:bool)
          n162 = xnode ("Discrete Delay")("D"=w294, "n-1[0..255]"=w281) -> ("Q"=w293:u64)
          n163 = xnode ("Discrete Delay")("D"=w299, "n-1[0..255]"=w281) -> ("Q"=w300:bool)
          n164 = xnode ("Discrete Delay")("D"=w310, "n-1[0..255]"=w270) -> ("Q"=w306:u64)
          n165 = xnode ("Discrete Delay")("D"=w309, "n-1[0..255]"=w270) -> ("Q"=w301:bool)
          n166 = Bundle("Q"=w301, "Q"=w300, "Q"=w297, "Q"=w295, "Q"=w267, "Q"=w286, "valid"=w272) -> (w271:T2)  [unwired: 1 in]
          n167 = Compound Arithmetic op=OR(w301, w300, w297, w295, w267, w286, w272) -> (w311:bool)
          n168 = Cluster To Array(cluster=w271) -> (array=w308:bool[])
          n169 = Boolean Array To Number(Boolean array=w308) -> (number=w307:u8)
          n170 = case shown="32" w307 {
            tunnel: [u64 0 ("out") w313 w314 w315 w316 w317 w318 w319] -> w305
            tunnel: w306 -> [_ w313 _ _ _ _ _ _]
            tunnel: w293 -> [_ _ w314 _ _ _ _ _]
            tunnel: w291 -> [_ _ _ w315 _ _ _ _]
            tunnel: w289 -> [_ _ _ _ w316 _ _ _]
            tunnel: w282 -> [_ _ _ _ _ w317 _ _]
            tunnel: w284 -> [_ _ _ _ _ _ w318 _]
            tunnel: w269 -> [_ _ _ _ _ _ _ w319]
            frame 0, Default {
            }
            frame 1 {
            }
            frame 2 {
            }
            frame 4 {
            }
            frame 8 {
            }
            frame 16 {
            }
            frame 32 {
            }
            frame 64 {
            }
          }
        }
        frame Disabled {
        }
      }
    }
    frame 13 {
      n171 = disable-structure shown="Enabled" {
        disable-tunnel: [w418 w525 _] -> w325
        disable-tunnel: [w413 w521 _] -> w324
        disable-tunnel: w323 -> [w348 w466 _]
        disable-tunnel: w322 -> [w347 w444 _]
        disable-tunnel: w321 -> [w346 w465 _]
        disable-tunnel: w320 -> [w334 w445 _]
        frame Disabled {
          n172 = Multiply(x=w334, y=u8 2 ("x")) -> (x*y=w335:u8)
          n173 = Multiply(x=w334, y=u8 11 ("x")) -> (x*y=w344:u8)
          n174 = Multiply(x=w334, y=u8 3 ("x")) -> (x*y=w336:u8)
          n175 = Multiply(x=w334, y=u8 10 ("x")) -> (x*y=w343:u8)
          n176 = Multiply(x=w334, y=u8 4 ("x")) -> (x*y=w337:u8)
          n177 = Multiply(x=w334, y=u8 8 ("x")) -> (x*y=w341:u8)
          n178 = Multiply(x=w334, y=u8 9 ("x")) -> (x*y=w342:u8)
          n179 = Multiply(x=w334, y=u8 5 ("x")) -> (x*y=w338:u8)
          n180 = Multiply(x=w334, y=u8 6 ("x")) -> (x*y=w339:u8)
          n181 = Multiply(x=w334, y=u8 7 ("x")) -> (x*y=w340:u8)
          n182 = Multiply(x=w334, y=u8 12 ("x")) -> (x*y=w384:u8)
          n183 = xnode ("Discrete Delay")("D"=w348, "n-1[0..255]"=w344) -> ("Q"=w350:u32)
          n184 = xnode ("Discrete Delay")("D"=w348, "n-1[0..255]"=w343) -> ("Q"=w357:u32)
          n185 = xnode ("Discrete Delay")("D"=w348, "n-1[0..255]"=w341) -> ("Q"=w363:u32)
          n186 = xnode ("Discrete Delay")("D"=w348, "n-1[0..255]"=w342) -> ("Q"=w360:u32)
          n187 = xnode ("Discrete Delay")("D"=w348, "n-1[0..255]"=w334) -> ("Q"=w417:u32)
          n188 = xnode ("Discrete Delay")("D"=w348, "n-1[0..255]"=w335) -> ("Q"=w411:u32)
          n189 = xnode ("Discrete Delay")("D"=w348, "n-1[0..255]"=w336) -> ("Q"=w409:u32)
          n190 = xnode ("Discrete Delay")("D"=w348, "n-1[0..255]"=w337) -> ("Q"=w407:u32)
          n191 = xnode ("Discrete Delay")("D"=w348, "n-1[0..255]"=w338) -> ("Q"=w393:u32)
          n192 = xnode ("Discrete Delay")("D"=w348, "n-1[0..255]"=w384) -> ("Q"=w385:u32)
          n193 = xnode ("Discrete Delay")("D"=w348, "n-1[0..255]"=w339) -> ("Q"=w378:u32)
          n194 = xnode ("Discrete Delay")("D"=w348, "n-1[0..255]"=w340) -> ("Q"=w368:u32)
          n195 = call "xcorr_packet_U64.vi"("x"=w347, "y"=w350, "trigger"=w346) -> ("out"=w326:u64, "valid"=w349:bool)  [unwired: 5 in]
          n196 = call "xcorr_packet_U64.vi"("x"=w347, "y"=w357, "trigger"=w346) -> ("out"=w327:u64, "valid"=w358:bool)  [unwired: 5 in]
          n197 = call "xcorr_packet_U64.vi"("x"=w347, "y"=w363, "trigger"=w346) -> ("out"=w365:u64, "valid"=w364:bool)  [unwired: 5 in]
          n198 = call "xcorr_packet_U64.vi"("x"=w347, "y"=w360, "trigger"=w346) -> ("out"=w328:u64, "valid"=w359:bool)  [unwired: 5 in]
          n199 = call "xcorr_packet_U64.vi"("x"=w347, "y"=w348, "trigger"=w346) -> ("out"=w416:u64, "valid"=w415:bool)  [unwired: 5 in]
          n200 = call "xcorr_packet_U64.vi"("x"=w347, "y"=w417, "trigger"=w346) -> ("out"=w399:u64, "valid"=w404:bool)  [unwired: 5 in]
          n201 = call "xcorr_packet_U64.vi"("x"=w347, "y"=w411, "trigger"=w346) -> ("out"=w398:u64, "valid"=w403:bool)  [unwired: 5 in]
          n202 = call "xcorr_packet_U64.vi"("x"=w347, "y"=w409, "trigger"=w346) -> ("out"=w396:u64, "valid"=w401:bool)  [unwired: 5 in]
          n203 = call "xcorr_packet_U64.vi"("x"=w347, "y"=w407, "trigger"=w346) -> ("out"=w388:u64, "valid"=w382:bool)  [unwired: 5 in]
          n204 = call "xcorr_packet_U64.vi"("x"=w347, "y"=w393, "trigger"=w346) -> ("out"=w390:u64, "valid"=w392:bool)  [unwired: 5 in]
          n205 = call "xcorr_packet_U64.vi"("x"=w347, "y"=w385, "trigger"=w346) -> ("out"=w383:u64, "valid"=w375:bool)  [unwired: 5 in]
          n206 = call "xcorr_packet_U64.vi"("x"=w347, "y"=w378, "trigger"=w346) -> ("out"=w380:u64, "valid"=w379:bool)  [unwired: 5 in]
          n207 = call "xcorr_packet_U64.vi"("x"=w347, "y"=w368, "trigger"=w346) -> ("out"=w366:u64, "valid"=w367:bool)  [unwired: 5 in]
          n208 = xnode ("Discrete Delay")("D"=w326, "n-1[0..255]"=w334) -> ("Q"=w330:u64)
          n209 = xnode ("Discrete Delay")("D"=w349, "n-1[0..255]"=w334) -> ("Q"=w345:bool)
          n210 = xnode ("Discrete Delay")("D"=w327, "n-1[0..255]"=w335) -> ("Q"=w331:u64)
          n211 = xnode ("Discrete Delay")("D"=w358, "n-1[0..255]"=w335) -> ("Q"=w352:bool)
          n212 = xnode ("Discrete Delay")("D"=w328, "n-1[0..255]"=w336) -> ("Q"=w332:u64)
          n213 = xnode ("Discrete Delay")("D"=w359, "n-1[0..255]"=w336) -> ("Q"=w353:bool)
          n214 = xnode ("Discrete Delay")("D"=w365, "n-1[0..255]"=w337) -> ("Q"=w333:u64)
          n215 = xnode ("Discrete Delay")("D"=w364, "n-1[0..255]"=w337) -> ("Q"=w354:bool)
          n216 = xnode ("Discrete Delay")("D"=w366, "n-1[0..255]"=w338) -> ("Q"=w329:u64)
          n217 = xnode ("Discrete Delay")("D"=w367, "n-1[0..255]"=w338) -> ("Q"=w355:bool)
          n218 = xnode ("Discrete Delay")("D"=w380, "n-1[0..255]"=w339) -> ("Q"=w376:u64)
          n219 = xnode ("Discrete Delay")("D"=w379, "n-1[0..255]"=w339) -> ("Q"=w373:bool)
          n220 = xnode ("Discrete Delay")("D"=w390, "n-1[0..255]"=w340) -> ("Q"=w389:u64)
          n221 = xnode ("Discrete Delay")("D"=w392, "n-1[0..255]"=w340) -> ("Q"=w391:bool)
          n222 = xnode ("Discrete Delay")("D"=w388, "n-1[0..255]"=w341) -> ("Q"=w387:u64)
          n223 = xnode ("Discrete Delay")("D"=w382, "n-1[0..255]"=w341) -> ("Q"=w381:bool)
          n224 = xnode ("Discrete Delay")("D"=w396, "n-1[0..255]"=w342) -> ("Q"=w395:u64)
          n225 = xnode ("Discrete Delay")("D"=w401, "n-1[0..255]"=w342) -> ("Q"=w400:bool)
          n226 = xnode ("Discrete Delay")("D"=w398, "n-1[0..255]"=w343) -> ("Q"=w397:u64)
          n227 = xnode ("Discrete Delay")("D"=w403, "n-1[0..255]"=w343) -> ("Q"=w402:bool)
          n228 = xnode ("Discrete Delay")("D"=w399, "n-1[0..255]"=w344) -> ("Q"=w374:u64)
          n229 = xnode ("Discrete Delay")("D"=w404, "n-1[0..255]"=w344) -> ("Q"=w405:bool)
          n230 = xnode ("Discrete Delay")("D"=w416, "n-1[0..255]"=w384) -> ("Q"=w414:u64)
          n231 = xnode ("Discrete Delay")("D"=w415, "n-1[0..255]"=w384) -> ("Q"=w406:bool)
          n232 = Bundle("Q"=w406, "Q"=w405, "Q"=w402, "Q"=w400, "Q"=w381, "Q"=w391, "Q"=w373, "Q"=w355, "Q"=w354, "Q"=w353, "Q"=w352, "Q"=w345, "valid"=w375) -> (w372:T3)  [unwired: 1 in]
          n233 = Compound Arithmetic op=OR(w406, w405, w402, w400, w381, w391, w373, w355, w354, w353, w352, w345, w375) -> (w418:bool)
          n234 = Cluster To Array(cluster=w372) -> (array=w370:bool[])
          n235 = Boolean Array To Number(Boolean array=w370) -> (number=w371:u16)
          n236 = case shown="0, Default" w371 {
            tunnel: [u64 0 ("out") w420 w421 w422 w423 w424 w425 w426 w427 w428 w429 w430 w431 w432] -> w413
            tunnel: w414 -> [_ w420 _ _ _ _ _ _ _ _ _ _ _ _]
            tunnel: w374 -> [_ _ w421 _ _ _ _ _ _ _ _ _ _ _]
            tunnel: w397 -> [_ _ _ w422 _ _ _ _ _ _ _ _ _ _]
            tunnel: w395 -> [_ _ _ _ w423 _ _ _ _ _ _ _ _ _]
            tunnel: w387 -> [_ _ _ _ _ w424 _ _ _ _ _ _ _ _]
            tunnel: w389 -> [_ _ _ _ _ _ w425 _ _ _ _ _ _ _]
            tunnel: w383 -> [_ _ _ _ _ _ _ _ _ _ _ _ _ w432]
            tunnel: w376 -> [_ _ _ _ _ _ _ w426 _ _ _ _ _ _]
            tunnel: w329 -> [_ _ _ _ _ _ _ _ w427 _ _ _ _ _]
            tunnel: w333 -> [_ _ _ _ _ _ _ _ _ w428 _ _ _ _]
            tunnel: w332 -> [_ _ _ _ _ _ _ _ _ _ w429 _ _ _]
            tunnel: w331 -> [_ _ _ _ _ _ _ _ _ _ _ w430 _ _]
            tunnel: w330 -> [_ _ _ _ _ _ _ _ _ _ _ _ w431 _]
            frame 0, Default {
            }
            frame 1 {
            }
            frame 2 {
            }
            frame 4 {
            }
            frame 8 {
            }
            frame 16 {
            }
            frame 32 {
            }
            frame 64 {
            }
            frame 128 {
            }
            frame 256 {
            }
            frame 512 {
            }
            frame 1024 {
            }
            frame 2048 {
            }
            frame 4096 {
            }
          }
        }
        frame Enabled {
          n237 = Multiply(x=w445, y=u8 2 ("x")) -> (x*y=w454:u8)
          n238 = Multiply(x=w445, y=u8 11 ("x")) -> (x*y=w463:u8)
          n239 = Multiply(x=w445, y=u8 3 ("x")) -> (x*y=w455:u8)
          n240 = Multiply(x=w445, y=u8 10 ("x")) -> (x*y=w462:u8)
          n241 = Multiply(x=w445, y=u8 4 ("x")) -> (x*y=w456:u8)
          n242 = Multiply(x=w445, y=u8 8 ("x")) -> (x*y=w460:u8)
          n243 = Multiply(x=w445, y=u8 9 ("x")) -> (x*y=w461:u8)
          n244 = Multiply(x=w445, y=u8 5 ("x")) -> (x*y=w457:u8)
          n245 = Multiply(x=w445, y=u8 6 ("x")) -> (x*y=w458:u8)
          n246 = Multiply(x=w445, y=u8 7 ("x")) -> (x*y=w459:u8)
          n247 = Multiply(x=w445, y=u8 12 ("x")) -> (x*y=w496:u8)
          n248 = xnode ("Discrete Delay")("D"=w466, "n-1[0..255]"=w445) -> ("Q"=w433:u32)
          n249 = xnode ("Discrete Delay")("D"=w433, "n-1[0..255]"=w445) -> ("Q"=w443:u32)
          n250 = xnode ("Discrete Delay")("D"=w443, "n-1[0..255]"=w445) -> ("Q"=w442:u32)
          n251 = xnode ("Discrete Delay")("D"=w442, "n-1[0..255]"=w445) -> ("Q"=w441:u32)
          n252 = xnode ("Discrete Delay")("D"=w441, "n-1[0..255]"=w445) -> ("Q"=w440:u32)
          n253 = xnode ("Discrete Delay")("D"=w440, "n-1[0..255]"=w445) -> ("Q"=w439:u32)
          n254 = xnode ("Discrete Delay")("D"=w439, "n-1[0..255]"=w445) -> ("Q"=w438:u32)
          n255 = xnode ("Discrete Delay")("D"=w438, "n-1[0..255]"=w445) -> ("Q"=w437:u32)
          n256 = xnode ("Discrete Delay")("D"=w437, "n-1[0..255]"=w445) -> ("Q"=w436:u32)
          n257 = xnode ("Discrete Delay")("D"=w436, "n-1[0..255]"=w445) -> ("Q"=w435:u32)
          n258 = xnode ("Discrete Delay")("D"=w435, "n-1[0..255]"=w445) -> ("Q"=w434:u32)
          n259 = xnode ("Discrete Delay")("D"=w434, "n-1[0..255]"=w445) -> ("Q"=w497:u32)
          n260 = call "xcorr_packet_U64.vi"("x"=w444, "y"=w434, "trigger"=w465) -> ("out"=w446:u64, "valid"=w467:bool)  [unwired: 5 in]
          n261 = call "xcorr_packet_U64.vi"("x"=w444, "y"=w435, "trigger"=w465) -> ("out"=w447:u64, "valid"=w474:bool)  [unwired: 5 in]
          n262 = call "xcorr_packet_U64.vi"("x"=w444, "y"=w437, "trigger"=w465) -> ("out"=w479:u64, "valid"=w478:bool)  [unwired: 5 in]
          n263 = call "xcorr_packet_U64.vi"("x"=w444, "y"=w436, "trigger"=w465) -> ("out"=w448:u64, "valid"=w475:bool)  [unwired: 5 in]
          n264 = call "xcorr_packet_U64.vi"("x"=w444, "y"=w466, "trigger"=w465) -> ("out"=w524:u64, "valid"=w523:bool)  [unwired: 5 in]
          n265 = call "xcorr_packet_U64.vi"("x"=w444, "y"=w433, "trigger"=w465) -> ("out"=w510:u64, "valid"=w515:bool)  [unwired: 5 in]
          n266 = call "xcorr_packet_U64.vi"("x"=w444, "y"=w443, "trigger"=w465) -> ("out"=w509:u64, "valid"=w514:bool)  [unwired: 5 in]
          n267 = call "xcorr_packet_U64.vi"("x"=w444, "y"=w442, "trigger"=w465) -> ("out"=w507:u64, "valid"=w512:bool)  [unwired: 5 in]
          n268 = call "xcorr_packet_U64.vi"("x"=w444, "y"=w441, "trigger"=w465) -> ("out"=w500:u64, "valid"=w494:bool)  [unwired: 5 in]
          n269 = call "xcorr_packet_U64.vi"("x"=w444, "y"=w440, "trigger"=w465) -> ("out"=w502:u64, "valid"=w504:bool)  [unwired: 5 in]
          n270 = call "xcorr_packet_U64.vi"("x"=w444, "y"=w497, "trigger"=w465) -> ("out"=w495:u64, "valid"=w488:bool)  [unwired: 5 in]
          n271 = call "xcorr_packet_U64.vi"("x"=w444, "y"=w439, "trigger"=w465) -> ("out"=w492:u64, "valid"=w491:bool)  [unwired: 5 in]
          n272 = call "xcorr_packet_U64.vi"("x"=w444, "y"=w438, "trigger"=w465) -> ("out"=w480:u64, "valid"=w481:bool)  [unwired: 5 in]
          n273 = xnode ("Discrete Delay")("D"=w446, "n-1[0..255]"=w445) -> ("Q"=w450:u64)
          n274 = xnode ("Discrete Delay")("D"=w467, "n-1[0..255]"=w445) -> ("Q"=w464:bool)
          n275 = xnode ("Discrete Delay")("D"=w447, "n-1[0..255]"=w454) -> ("Q"=w451:u64)
          n276 = xnode ("Discrete Delay")("D"=w474, "n-1[0..255]"=w454) -> ("Q"=w469:bool)
          n277 = xnode ("Discrete Delay")("D"=w448, "n-1[0..255]"=w455) -> ("Q"=w452:u64)
          n278 = xnode ("Discrete Delay")("D"=w475, "n-1[0..255]"=w455) -> ("Q"=w470:bool)
          n279 = xnode ("Discrete Delay")("D"=w479, "n-1[0..255]"=w456) -> ("Q"=w453:u64)
          n280 = xnode ("Discrete Delay")("D"=w478, "n-1[0..255]"=w456) -> ("Q"=w471:bool)
          n281 = xnode ("Discrete Delay")("D"=w480, "n-1[0..255]"=w457) -> ("Q"=w449:u64)
          n282 = xnode ("Discrete Delay")("D"=w481, "n-1[0..255]"=w457) -> ("Q"=w472:bool)
          n283 = xnode ("Discrete Delay")("D"=w492, "n-1[0..255]"=w458) -> ("Q"=w489:u64)
          n284 = xnode ("Discrete Delay")("D"=w491, "n-1[0..255]"=w458) -> ("Q"=w486:bool)
          n285 = xnode ("Discrete Delay")("D"=w502, "n-1[0..255]"=w459) -> ("Q"=w501:u64)
          n286 = xnode ("Discrete Delay")("D"=w504, "n-1[0..255]"=w459) -> ("Q"=w503:bool)
          n287 = xnode ("Discrete Delay")("D"=w500, "n-1[0..255]"=w460) -> ("Q"=w499:u64)
          n288 = xnode ("Discrete Delay")("D"=w494, "n-1[0..255]"=w460) -> ("Q"=w493:bool)
          n289 = xnode ("Discrete Delay")("D"=w507, "n-1[0..255]"=w461) -> ("Q"=w506:u64)
          n290 = xnode ("Discrete Delay")("D"=w512, "n-1[0..255]"=w461) -> ("Q"=w511:bool)
          n291 = xnode ("Discrete Delay")("D"=w509, "n-1[0..255]"=w462) -> ("Q"=w508:u64)
          n292 = xnode ("Discrete Delay")("D"=w514, "n-1[0..255]"=w462) -> ("Q"=w513:bool)
          n293 = xnode ("Discrete Delay")("D"=w510, "n-1[0..255]"=w463) -> ("Q"=w487:u64)
          n294 = xnode ("Discrete Delay")("D"=w515, "n-1[0..255]"=w463) -> ("Q"=w516:bool)
          n295 = xnode ("Discrete Delay")("D"=w524, "n-1[0..255]"=w496) -> ("Q"=w522:u64)
          n296 = xnode ("Discrete Delay")("D"=w523, "n-1[0..255]"=w496) -> ("Q"=w517:bool)
          n297 = Bundle("Q"=w517, "Q"=w516, "Q"=w513, "Q"=w511, "Q"=w493, "Q"=w503, "Q"=w486, "Q"=w472, "Q"=w471, "Q"=w470, "Q"=w469, "Q"=w464, "valid"=w488) -> (w485:T3)  [unwired: 1 in]
          n298 = Compound Arithmetic op=OR(w517, w516, w513, w511, w493, w503, w486, w472, w471, w470, w469, w464, w488) -> (w525:bool)
          n299 = Cluster To Array(cluster=w485) -> (array=w483:bool[])
          n300 = Boolean Array To Number(Boolean array=w483) -> (number=w484:u16)
          n301 = case shown="0, Default" w484 {
            tunnel: [u64 0 ("out") w527 w528 w529 w530 w531 w532 w533 w534 w535 w536 w537 w538 w539] -> w521
            tunnel: w522 -> [_ w527 _ _ _ _ _ _ _ _ _ _ _ _]
            tunnel: w487 -> [_ _ w528 _ _ _ _ _ _ _ _ _ _ _]
            tunnel: w508 -> [_ _ _ w529 _ _ _ _ _ _ _ _ _ _]
            tunnel: w506 -> [_ _ _ _ w530 _ _ _ _ _ _ _ _ _]
            tunnel: w499 -> [_ _ _ _ _ w531 _ _ _ _ _ _ _ _]
            tunnel: w501 -> [_ _ _ _ _ _ w532 _ _ _ _ _ _ _]
            tunnel: w495 -> [_ _ _ _ _ _ _ _ _ _ _ _ _ w539]
            tunnel: w489 -> [_ _ _ _ _ _ _ w533 _ _ _ _ _ _]
            tunnel: w449 -> [_ _ _ _ _ _ _ _ w534 _ _ _ _ _]
            tunnel: w453 -> [_ _ _ _ _ _ _ _ _ w535 _ _ _ _]
            tunnel: w452 -> [_ _ _ _ _ _ _ _ _ _ w536 _ _ _]
            tunnel: w451 -> [_ _ _ _ _ _ _ _ _ _ _ w537 _ _]
            tunnel: w450 -> [_ _ _ _ _ _ _ _ _ _ _ _ w538 _]
            frame 0, Default {
            }
            frame 1 {
            }
            frame 2 {
            }
            frame 4 {
            }
            frame 8 {
            }
            frame 16 {
            }
            frame 32 {
            }
            frame 64 {
            }
            frame 128 {
            }
            frame 256 {
            }
            frame 512 {
            }
            frame 1024 {
            }
            frame 2048 {
            }
            frame 4096 {
            }
          }
        }
        frame Disabled {
        }
      }
    }
  }
  "trigger" <- w12
  "Rxy valid" <- w13
  "Rxy" <- w7
